vi "RobotMap.vi"() -> ()   [LabVIEW 2018]
panel:
  in  "RightDriveSlave":u8=4
  in  "RightDriveMaster":u8=3
  in  "LeftDriveSlave":u8=2
  in  "LeftDriveMaster":u8=1
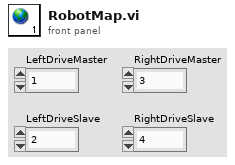
[diagram p1: front panel]
diagram:
